vi "builder main.vi"(8 "error in (no error)":errorcluster, 10 "builder settings":T1, 11 "CLI":refnum<class "CLI.lvclass">) -> (0 "error out":errorcluster, 2 "Destinations":T2[](array[typedef]), 3 "GeneratedFiles":path[](array[path]))   [LabVIEW 2024]
uses:
  builders/parent/Builder.lvclass
  <vilib>/AppBuilder/AB_API/common/AB_API Destination Type.ctl
  <vilib>/AppBuilder/AB_API/common/AB_API Destination Data.ctl
  builders/parent/builder settings.ctl
  <vilib>/Wiresmith Technology/G CLI/CLI Class/CLI.lvclass
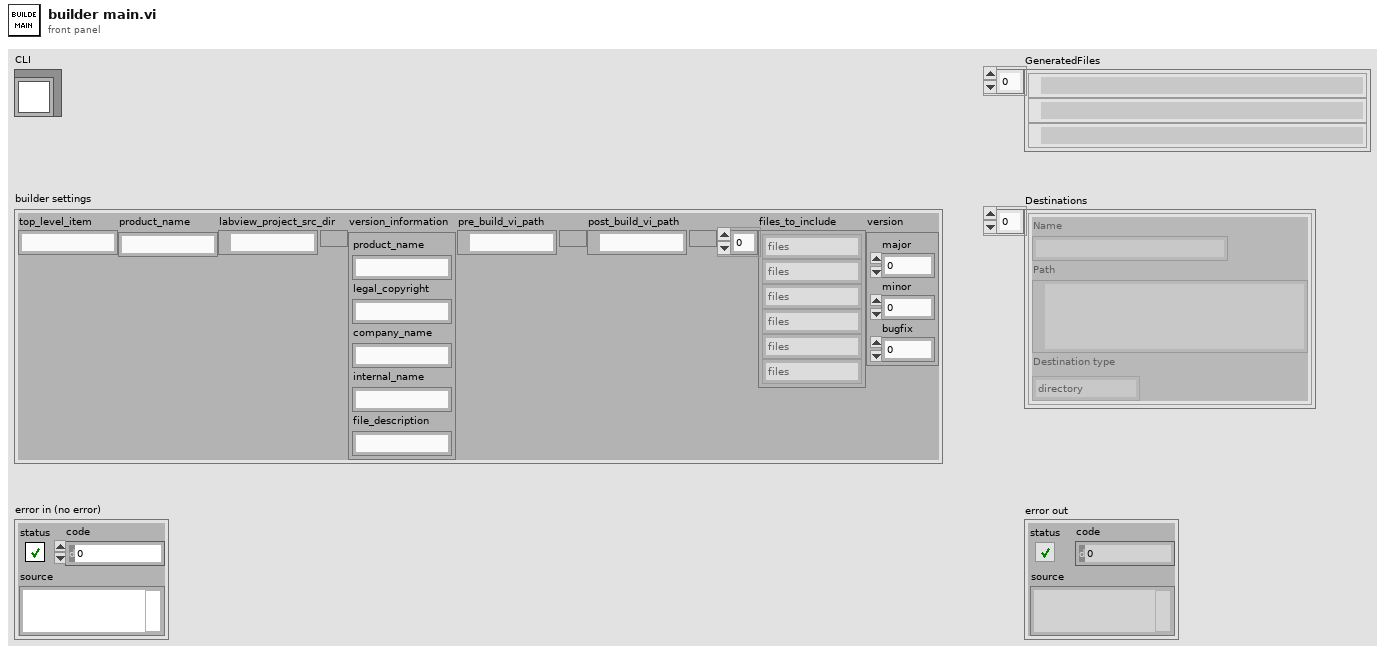
[diagram p1: front panel]
types:
  T1 = typedef "Builder.lvclass/builder settings.ctl" = cluster{"top_level_item":string, "product_name":string, "labview_project_src_dir":path, "version_information":cluster{"product_name":string, "legal_copyright":string, "company_name":string, "internal_name":string, "file_description":string}, "pre_build_vi_path":path, "post_build_vi_path":path, "files_to_include":string[], "version":cluster{"major":u16, "minor":u16, "bugfix":u16}}
  T2 = typedef "AB_API Destination Data.ctl" = cluster{"Name":string, "Path":path, "Destination type":T3}
  T3 = typedef "AB_API Destination Type.ctl" = enum16{"directory", "directory (preserve hierarchy)", "LLB"}
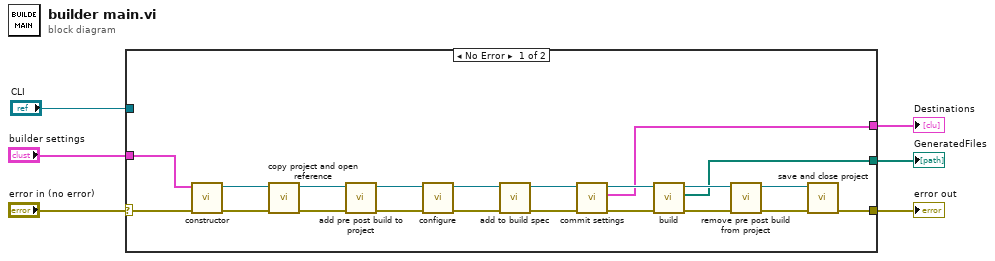
[diagram p0: block diagram]
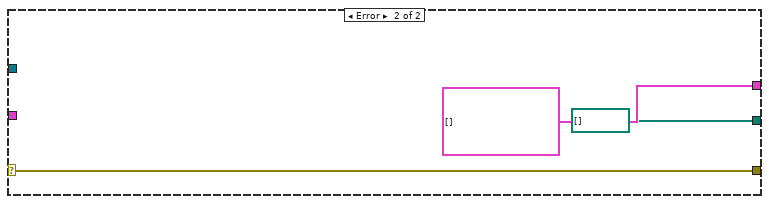
[diagram p2: hidden frame]
diagram:
  n1 = case shown="No Error" "error in (no error)" {
    selector: "error in (no error)" -> [w24 w30]
    tunnel: [w10 path[] [] ("GeneratedFiles")] -> w2
    tunnel: [w7 T2[] [] ("Destinations")] -> w6
    tunnel: [w12 w30] -> w5
    tunnel: "builder settings" -> [w8 _]
    tunnel: "CLI" -> [_ _]
    frame No Error {
      n2 = call "constructor.vi"("error in (no error)"=w24, "builder settings"=w8) -> ("error out"=w23:errorcluster, "Builders"=w9:refnum<class "Builder.lvclass">)  [unwired: 8 in]
      n3 = call "copy project and open reference.vi"("error in (no error)"=w23, "Builder in"=w9) -> ("error out"=w25:errorcluster, "Builder out"=w26:refnum<class "Builder.lvclass">)  [unwired: 8 in]
      n4 = call "add pre post build to project.vi"("error in (no error)"=w25, "Builder"=w26) -> ("error out"=w19:errorcluster, "Builder out"=w22:refnum<class "Builder.lvclass">)  [unwired: 8 in]
      n5 = call-dynamic "configure.vi"("error in (no error)"=w19, "Builders in"=w22) -> ("error out"=w20:errorcluster, "Builders out"=w21:refnum<class "Builder.lvclass">)  [unwired: 8 in]
      n6 = call-dynamic "add to build spec.vi"("error in (no error)"=w20, "Builders in"=w21) -> ("error out"=w18:errorcluster, "Builders out"=w17:refnum<class "Builder.lvclass">)  [unwired: 8 in]
      n7 = call-dynamic "commit settings.vi"("error in (no error)"=w18, "Builders in"=w17) -> ("error out"=w15:errorcluster, "Destinations"=w7:T2[], "Builders out"=w16:refnum<class "Builder.lvclass">)  [unwired: 7 in]
      n8 = call-dynamic "build.vi"("error in (no error)"=w15, "Builder in"=w16) -> ("error out"=w13:errorcluster, "GeneratedFiles"=w10:path[], "Builder out"=w14:refnum<class "Builder.lvclass">)  [unwired: 7 in]
      n9 = call "remove pre post build from project.vi"("error in (no error)"=w13, "Builder in"=w14) -> ("error out"=w27:errorcluster, "Builder out"=w11:refnum<class "Builder.lvclass">)  [unwired: 8 in]
      n10 = call "save and close project.vi"("error in (no error)"=w27, "Builders.lvclass"=w11) -> ("error out"=w12:errorcluster)  [unwired: 9 in]
    }
    frame Error {
    }
  }
  "Destinations" <- w6
  "error out" <- w5
  "GeneratedFiles" <- w2
